vi "Creators Created Queues.vi"(8 "Created Queue Alias":string, 9 "Priority?":bool, 10 "Msg Strategy":refnum<class "Msg Strategy.lvclass">, 11 "Base Event jettl in":refnum<class "Base Event jettl.lvclass">) -> (3 "Base Event jettl out":refnum<class "Base Event jettl.lvclass">)   [LabVIEW 2021, in "jettl.lvlib" / "Base Event jettl.lvlib" / "Base Event jettl.lvclass"]
uses:
  Base Event jettl.lvclass
  Queue Mailbox/Queue Mailbox.lvlib
  Msg Strategy/Msg Strategy.lvclass
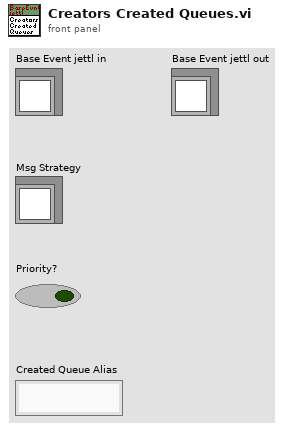
[diagram p1: front panel]
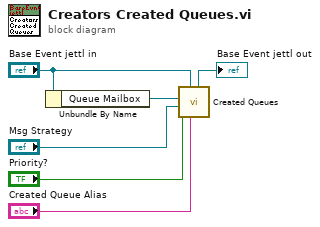
[diagram p0: block diagram]
diagram:
  n1 = Unbundle By Name("Base Event jettl in") -> ("Queue Mailbox"=w6:refnum<data-value>)
  n2 = call "Created Queues.vi"("Created Queue Alias"="Created Queue Alias", "jettl in"="Base Event jettl in", "Priority?"="Priority?", "Msg Strategy"="Msg Strategy", "Queue Mailbox"=w6) -> ("jettl out"=→"Base Event jettl out":refnum<class "Base Event jettl.lvclass">)  [unwired: 6 in]
